vi "ADsinMerge.vi"(8 "tol":dbl=0.2, 9 "Encoder Position":i32, 11 "Cos Sin Input":dbl[](array[numeric])) -> (0 "Tolerance Fail Count":u16, 3 "Final Position":dbl)   [LabVIEW 2010, in "kevLib2010.lvlib"]
uses:
  kevLib2010.lvlib
panel:
  # "This function REQUIRES the cos sine to align correctly with the signs of the encoder\nWhat are they? I forgot :-P"
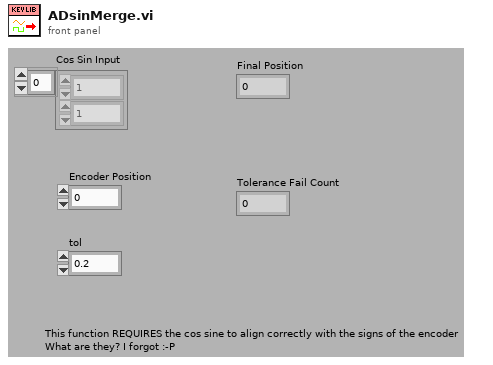
[diagram p1: front panel]
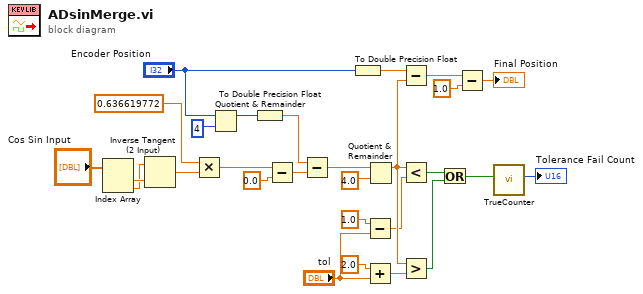
[diagram p0: block diagram]
diagram:
  n1 = Index Array(array="Cos Sin Input") -> (element #1=w2:dbl, element #2=w1:dbl)  [unwired: 2 in]
  n2 = Inverse Tangent (2 Input)(1:w2, 2:w1) -> (0:w6:dbl)
  n3 = Multiply(x=0.636619772, y=w6) -> (x*y=w10:dbl)
  n4 = Quotient & Remainder(x="Encoder Position", y=4) -> (x-y*floor(x/y)=w9:i32)  [unwired: 1 out]
  n5 = To Double Precision Float(number=w9) -> (double precision float=w22:dbl)
  n6 = Subtract(x=w10, y=0.0) -> (x-y=w13:dbl)
  n7 = Subtract(x=w22, y=w13) -> (x-y=w14:dbl)
  n8 = To Double Precision Float(number="Encoder Position") -> (double precision float=w24:dbl)
  n9 = Subtract(x=1.0 ("y"), y="tol") -> (x-y=w16:dbl)
  n10 = Add(x=2.0 ("y"), y="tol") -> (x+y=w19:dbl)
  n11 = Quotient & Remainder(x=w14, y=4.0) -> (x-y*floor(x/y)=w25:dbl)  [unwired: 1 out]
  n12 = Subtract(x=w24, y=w25) -> (x-y=w26:dbl)
  n13 = Less?(x=w25, y=w16) -> (x < y?=w21:bool)
  n14 = Greater?(x=w25, y=w19) -> (0:w20:bool)
  n15 = Or(x=w21, y=w20) -> (x .or. y?=w5:bool)
  n16 = Subtract(x=w26, y=1.0) -> (x-y=→"Final Position":dbl)
  n17 = call "TrueCounter.vi"("True?"=w5) -> ("True Count"=→"Tolerance Fail Count":u16)  [unwired: 9 in]
